vi "labview_client.vi"() -> ()   [LabVIEW 2018]
doc: "You can use the System Exec VI to call command line utilities that return standard output to the command shell. You also can call interactive applications that you intend to launch using System Exec, but interact with using the UI of the executable."
panel:
  out "standard output":string
  out "standard error":string
  out "return code":i32
  # "Overview: Client that receives data from server\nRequirements: Windows"
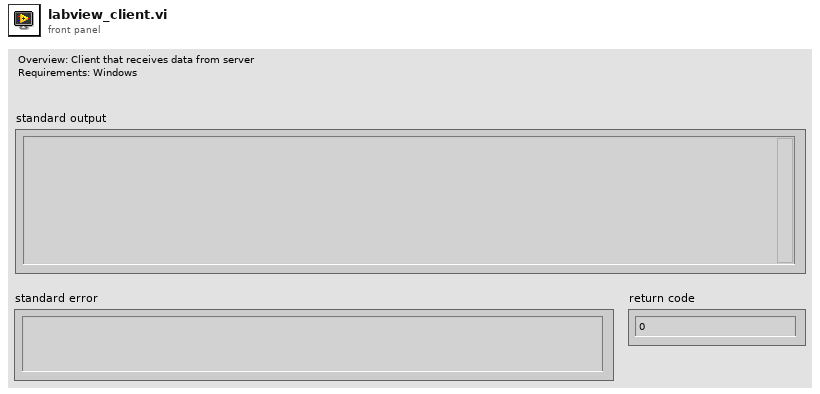
[diagram p1: front panel]
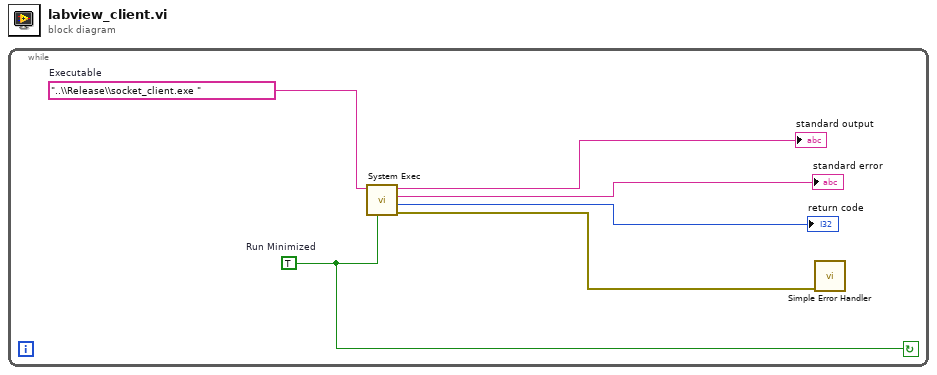
[diagram p0: block diagram]
diagram:
  n1 = while {
    stop <- w2 continue-if-true
    w2 = TRUE  # Run Minimized
    w6 = "..\\Release\\socket_client.exe "  # Executable
    n2 = call <vilib>:"System Exec.vi"("run minimized? (F)"=w2, "command line"=w6) -> ("error out"=w3:errorcluster, "return code"=→"return code":i32, "standard error"=→"standard error":string, "standard output"=→"standard output":string)  [unwired: 6 in]
    n3 = call <vilib>:"Simple Error Handler.vi"("error in (no error)"=w3) -> ()  [unwired: 1 in, 8 out]
  }
